vi "Write-Read from Instrument.vi"(8 "error in (no error)":errorcluster, 9 "Value to Send":dbl, 10 "Address":string, 11 "heater_parent in":refnum<class "heater_parent.lvclass">) -> (0 "error out":errorcluster, 2 "Value Read":dbl, 3 "heater_parent out":refnum<class "heater_parent.lvclass">)   [LabVIEW 2020, in "polar_bear_plus_drivers.lvlib" / "heater_parent.lvclass"]
doc: "Write a command, wait to give the instrument adequate time to respond, and read the response."
uses:
  <instrlib>/RxnRover/Driver Polar Bear Plus/heater_parent/heater_parent.lvclass
  <instrlib>/RxnRover/Driver Polar Bear Plus/heater_parent/heater_parent.lvclass/heater_parent.ctl
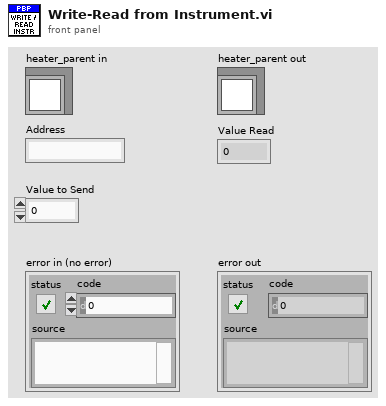
[diagram p1: front panel]
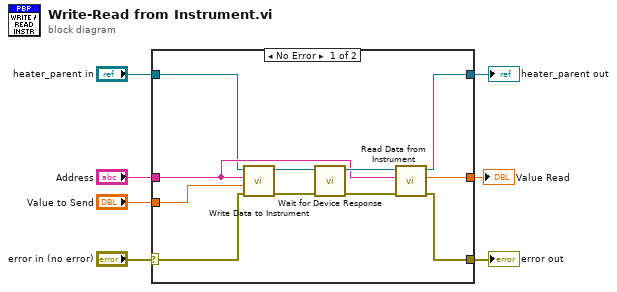
[diagram p0: block diagram]
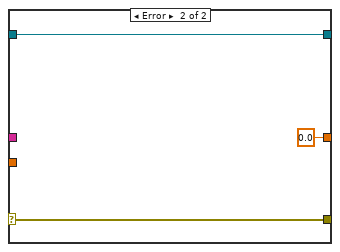
[diagram p2: hidden frame]
diagram:
  n1 = case shown="No Error" "error in (no error)" {
    selector: "error in (no error)" -> [w10 w20]
    tunnel: [w12 w21] -> w7
    tunnel: [w9 w20] -> w6
    tunnel: "heater_parent in" -> [w13 w21]
    tunnel: [w11 0.0 ("Value Read")] -> w2
    tunnel: "Address" -> [w14 _]
    tunnel: "Value to Send" -> [w8 _]
    frame No Error {
      n2 = call-dynamic "Write Data to Instrument.vi"("error in (no error)"=w10, "Value to Send"=w8, "Address"=w14, "heater_parent in"=w13) -> ("error out"=w18:errorcluster, "heater_parent out"=w16:refnum<class "heater_parent.lvclass">)  [unwired: 6 in]
      n3 = call-dynamic "Wait for Device Response.vi"("error in (no error)"=w18, "heater_parent in"=w16) -> ("error out"=w17:errorcluster, "heater_parent out"=w15:refnum<class "heater_parent.lvclass">)  [unwired: 8 in]
      n4 = call-dynamic "Read Data from Instrument.vi"("error in (no error)"=w17, "Address"=w14, "heater_parent in"=w15) -> ("error out"=w9:errorcluster, "Value Read"=w11:dbl, "heater_parent out"=w12:refnum<class "heater_parent.lvclass">)  [unwired: 6 in]
    }
    frame Error {
    }
  }
  "heater_parent out" <- w7
  "error out" <- w6
  "Value Read" <- w2
